vi "ReadDigitalOutput.vi"(8 "error in (no error)":errorcluster, 11 "TesteractHAL_DigitalOutput_NIDAQmx In":refnum<class "TesteractHAL_DigitalOutput_NIDAQmx.lvclass">) -> (0 "error out":errorcluster, 1 "Tristate":bool, 2 "data":bool, 3 "TesteractHAL_DigitalOutput_NIDAQmx Out":refnum<class "TesteractHAL_DigitalOutput_NIDAQmx.lvclass">)   [LabVIEW 2017, in "TesteractHAL_DigitalOutput_NIDAQmx.lvlib" / "TesteractHAL_DigitalOutput_NIDAQmx.lvclass"]
doc: "Read a single line"
uses:
  TesteractHAL_DigitalOutput_NIDAQmx.lvclass
  TesteractHAL_DigitalOutput_NIDAQmx.lvclass/TesteractHAL_DigitalOutput_NIDAQmx.ctl
  <vilib>/DAQmx/read.llb/DAQmx Read (Digital Bool 1Line 1Point).vi
  <vilib>/DAQmx/miscellaneous.llb/DAQmx Fill In Error Info.vi
  <resource>/objmgr/daqmx.rc
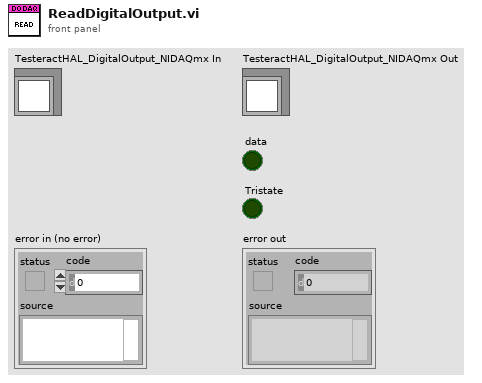
[diagram p1: front panel]
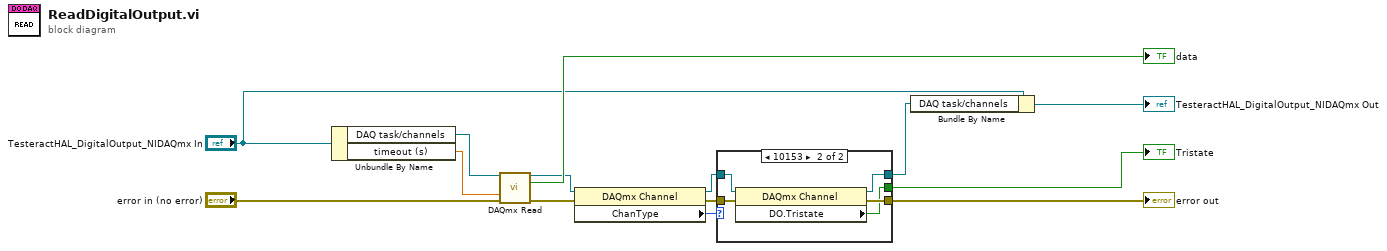
[diagram p0: block diagram]
diagram:
  n1 = Unbundle By Name("TesteractHAL_DigitalOutput_NIDAQmx In") -> ("DAQ task/channels"=w14:refnum<k21>, "timeout (s)"=w13:dbl)
  n2 = call-poly <vilib>:"DAQmx Read.vi"("task/channels in"=w14, "timeout"=w13, "error in"="error in (no error)") -> ("task out"=w7:refnum<k21>, "data"=→"data":bool, "error out"=w8:errorcluster)  [unwired: 10 in]
  n3 = property class="DAQmx Channel"(reference=w7, error in=w8) -> (reference out=w5:refnum<k21>, error out=w4:errorcluster, "ChanType"=w6:i32)
  n4 = case shown="10153" w6 {
    tunnel: w5 -> [w15 w21]
    tunnel: w4 -> [w16 w20]
    tunnel: [w15 w19] -> w3
    tunnel: [w16 w18] -> w2
    tunnel: [_ w17] -> w1
    frame Default {
    }
    frame 10153 {
      n5 = property class="DAQmx Channel"(reference=w21, error in=w20) -> (reference out=w19:refnum<k21>, error out=w18:errorcluster, "DO.Tristate"=w17:bool)
    }
  }
  "error out" <- w2
  "Tristate" <- w1
  n6 = Bundle By Name(cluster="TesteractHAL_DigitalOutput_NIDAQmx In", "DAQ task/channels"=w3) -> (→"TesteractHAL_DigitalOutput_NIDAQmx Out":refnum<class "TesteractHAL_DigitalOutput_NIDAQmx.lvclass">)
